vi "AddConnection.vi"(3 "String in":string, 5 "data":T3={"New Subscriber"={"Caller ID"="", "Topic Name"="", "Protocol"="", "URIs"="", "ID"=refnum}, "ROS of Server"={"topic port"=0, "Node"="", "topic"="", "type"="", "node port"=0, "error "={"status"=FALSE, "code"=0, "source"=""}, "Direction"=enum."Node", "APIs"=[], "Update (ms)"=1, "write queue"=1}, "new port"=0}) -> (0 "String out":string, 1 "Log":T2, 2 "MyState":T1)   [LabVIEW 2012]
uses:
  SubVIs/_ROSDirection.ctl
  SubVIs/_ROSControl.ctl
  requestTopic.ctl
  ROSLog.ctl
  MyState.ctl
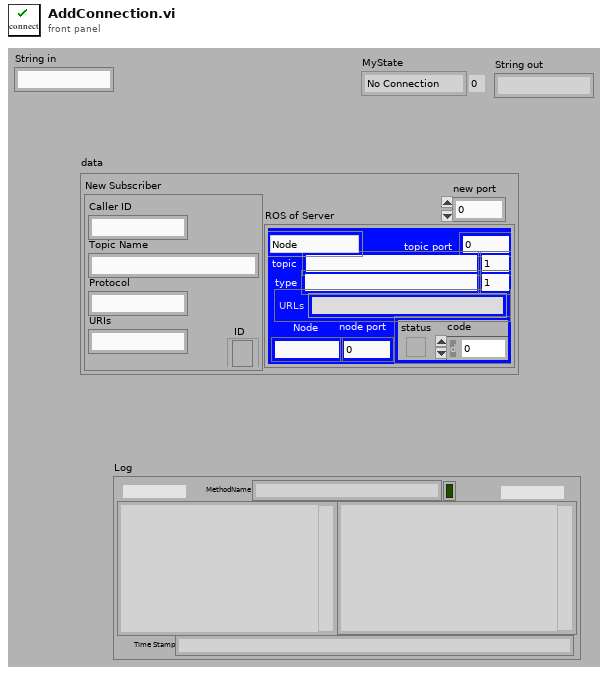
[diagram p1: front panel]
types:
  T1 = typedef "MyState.ctl" = enum16{"No Connection", "Registered", "Connected", "Close"}
  T2 = typedef "ROSLog.ctl" = cluster{"Sent":string, "Reply":string, "MethodName":string, "success":bool, "Dir1":string, "Dir2":string, "Time Stamp":string}
  T3 = typedef "requestTopic.ctl" = cluster{"New Subscriber":cluster{"Caller ID":string, "Topic Name":string, "Protocol":string, "URIs":string, "ID":refnum<k5>}, "ROS of Server":T4, "new port":u16}
  T4 = typedef "_ROSControl.ctl" = cluster{"topic port":u16, "Node":string, "topic":string, "type":string, "node port":u32, "error ":errorcluster, "Direction":T5, "APIs":string[], "Update (ms)":u16, "write queue":u16}
  T5 = typedef "_ROSDirection.ctl" = enum16{"Node", "Publisher", "Subscriber", "Service Client"}
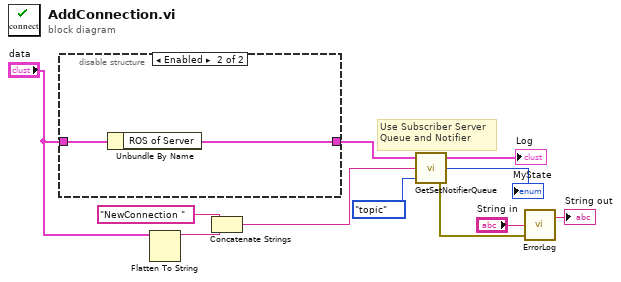
[diagram p0: block diagram]
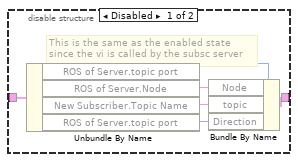
[diagram p2: hidden frame]
diagram:
  # "Use Subscriber Server \nQueue and Notifier"
  n1 = disable-structure shown="Enabled" {
    disable-tunnel: "data" -> [w14 w19]
    disable-tunnel: [w12 w18] -> w1
    frame Disabled {
      # "This is the same as the enabled state\nsince the vi is called by the subsc server"
      n2 = Unbundle By Name(w14) -> ("ROS of Server.topic port"=w13:u16, "ROS of Server.Node"=w15:string, "New Subscriber.Topic Name"=w17:string, "ROS of Server.topic port"=w16:u16)
      n3 = Bundle By Name(cluster=w13, "Node"=w15, "topic"=w17, "Direction"=w16) -> (w12:cluster{})
    }
    frame Enabled {
      n4 = Unbundle By Name(w19) -> ("ROS of Server"=w18:T4)
    }
  }
  n5 = Flatten To String(anything="data") -> (data string=w11:string)  [unwired: 3 in, 2 out]
  n6 = Concatenate Strings("NewConnection " ("element"), w11) -> (w8:string)
  n7 = call "GetSetNotifierQueue.vi"("Name"=enum16{"topic", "node"}."topic", "Command"=w8, "ROS"=w1) -> ("error out"=w5:errorcluster, "MyState"=→"MyState":T1, "Log"=→"Log":T2)
  n8 = call "ErrorLog.vi"("error in"=w5, "String in"="String in") -> ("String out"=→"String out":string)  [unwired: 1 in, 1 out]
